vi "MainFSM.vi"() -> ()   [LabVIEW 2017]
uses:
  States.ctl
  <extravilib>/ChannelInstances/Tag-bool/Read With Abort.vi
  <extravilib>/ChannelInstances/Tag-bool/Write With Abort.vi
  <extravilib>/ChannelInstances/Tag-bool/Instantiate.vi
  <extravilib>/ChannelInstances/Tag-bool/EndpointRead.vi
  <extravilib>/ChannelInstances/Tag-bool/Endpoint.vi
  <extravilib>/ChannelInstances/Tag-bool.lvlib
panel:
  out "State FSM 2":T1
  out "State FSM 1":T1
  in  "stop":bool
  in  "Command":bool
  # "Test Finite State Machine"
  # "Getestet wird FSM.vi\n\n1) FSM ist  \"Preallocated Reentrant\" (d.h. zwei FSM laufen unabhängig)\n2) FSM hat einen \"Init\" und einen \"Run\" state. In \"Init\" wird ein default\n     State gesetzt oder der Eingangswert wird gesetzt.\n3) In der oberen While-Loop wird im Timeout FSM per VI Server aufgerufen.\n\nVorsicht, das VI läuft nicht auf myRIO, da eine Event-Loop benutzt wird."
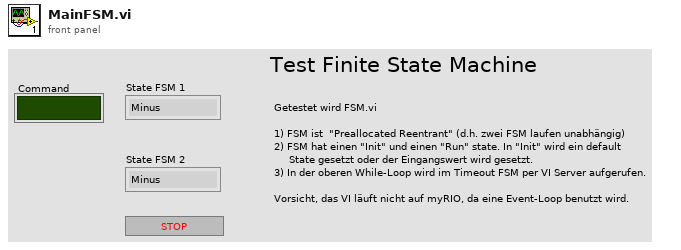
[diagram p1: front panel]
types:
  T1 = typedef "States.ctl" = enum16{"Minus", "Zero", "Plus"}
  T2 = typedef "Tag-bool.lvlib/))Channel.ctl" = refnum<queue>
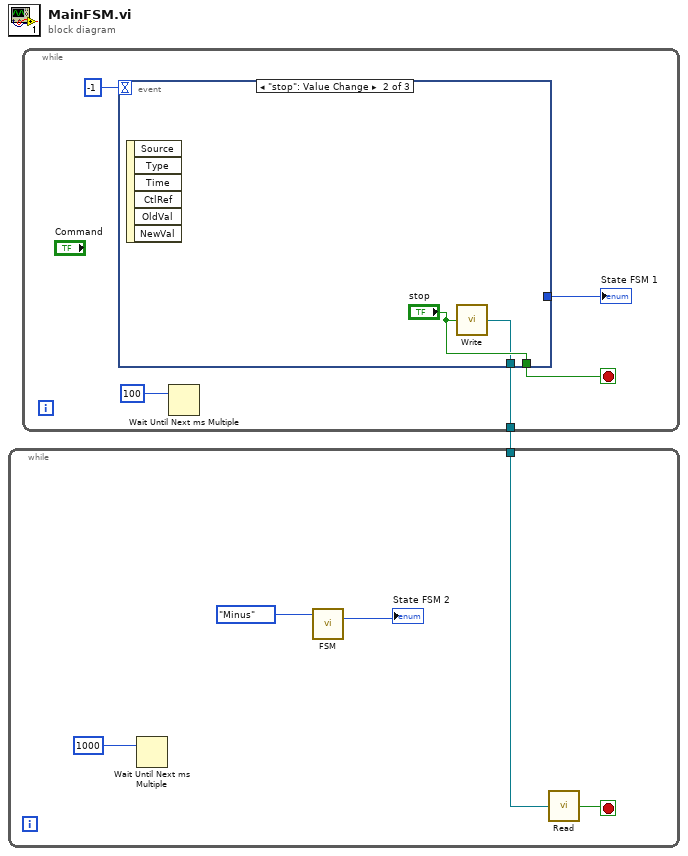
[diagram p0: block diagram]
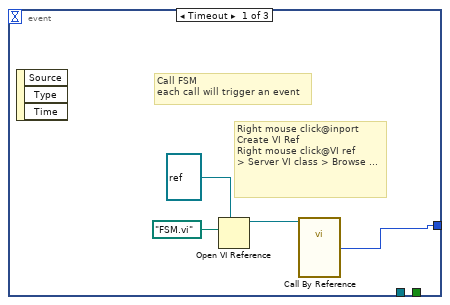
[diagram p2: hidden frame]
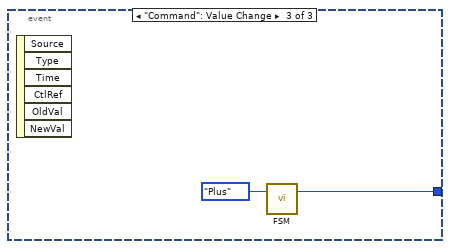
[diagram p3: hidden frame]
diagram:
  n1 = while {
    tunnel: [w2] -> w1
    stop <- w3 stop-if-true
    n2 = event shown="[1] \"stop\": Value Change" {
      selector: _ -> [_ _ _]
      dyn-events: _ -> [_ _ _]
      timeout: -1 -> [_ _ _]
      tunnel: [_ "stop" _] -> w3
      tunnel: [w10 _ w14] -> w5
      tunnel: [_ w11 _] -> w2
      event Timeout {
        # "Right mouse click@inport\nCreate VI Ref\nRight mouse click@VI ref\n> Server VI class > Browse ..."
        # "Call FSM\neach call will trigger an event"
        n3 = event-data() -> ()  [unwired: 1 in, 3 out]
        n4 = Open VI Reference(type specifier VI Refnum (for type only)=refnum<vi> refnum, vi path=path "FSM.vi") -> (vi reference=w7:refnum<vi>)  [unwired: 4 in, 1 out]
        n5 = call-by-ref "?"(reference=w7) -> ("Current\nState"=w10:T1)  [unwired: 4 in, 2 out]
      }
      event "stop": Value Change {
        n6 = event-data() -> ()  [unwired: 1 in, 6 out]
        n7 = call <extravilib>:"Write.vi"("element"="stop") -> ("channel"=w11:T2)  [unwired: 1 out]
      }
      event "Command": Value Change {
        n8 = event-data() -> ()  [unwired: 1 in, 6 out]
        n9 = call "FSM.vi"("Init State"=States."Plus") -> ("Current\nState"=w14:T1)  [unwired: 2 in]
      }
    }
    "State FSM 1" <- w5
    n10 = Wait Until Next ms Multiple(millisecond multiple=100) -> ()  [unwired: 1 out]
  }
  n11 = while {
    tunnel: w1 -> [w16]
    stop <- w15 stop-if-true
    n12 = Wait Until Next ms Multiple(millisecond multiple=1000) -> ()  [unwired: 1 out]
    n13 = call "FSM.vi"("Init State"=States."Minus") -> ("Current\nState"=→"State FSM 2":T1)  [unwired: 2 in]
    n14 = call <extravilib>:"Read.vi"("channel"=w16) -> ("element"=w15:bool)  [unwired: 1 in, 1 out]
  }
